vi "Initialize Variables.vi"(5 "subkey":string="Software\\DuPont\\BIMS", 6 "errorIN":errorcluster, 9 "InitCluster":cluster{"deployment":refnum<vi>}) -> (0 "errorOUT":errorcluster)   [LabVIEW 2010]
uses:
  <vilib>/registry/registry.llb/Registry SAM.ctl
  <vilib>/registry/registry.llb/Registry RtKey.ctl
panel:
  in  "DataFolder":refnum<vi>
  in  "Keys":enum16{"Root"}(ring)
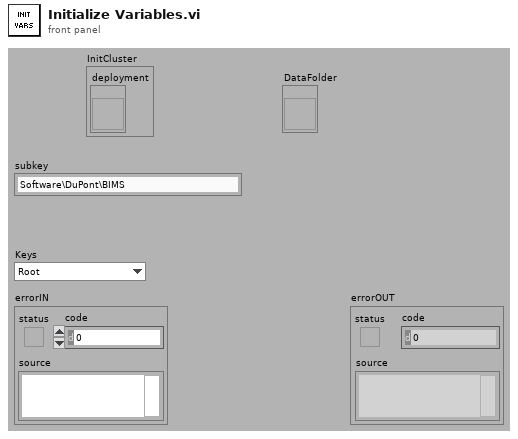
[diagram p1: front panel]
types:
  T1 = typedef "Registry SAM.ctl" = enum32{"KEY_QUERY_VALUE", "KEY_SET_VALUE", "KEY_CREATE_SUB_KEY", "KEY_ENUMERATE_SUB_KEYS", "KEY_NOTIFY", "KEY_CREATE_LINK", "KEY_READ", "KEY_WRITE", "KEY_ALL_ACCESS", "KEY_READ | KEY_WRITE"}
  T2 = typedef "Registry RtKey.ctl" = enum32{"HKEY_CLASSES_ROOT", "HKEY_CURRENT_USER", "HKEY_LOCAL_MACHINE", "HKEY_USERS", "HKEY_PERFORMANCE_DATA", "HKEY_CURRENT_CONFIG", "HKEY_DYN_DATA"}
  T3 = typedef "Registry refnum.ctl" = refnum<k1>
  T4 = cluster{"numValues":i32, "maxValueNameLen":i32, "maxValueDataLen":i32}
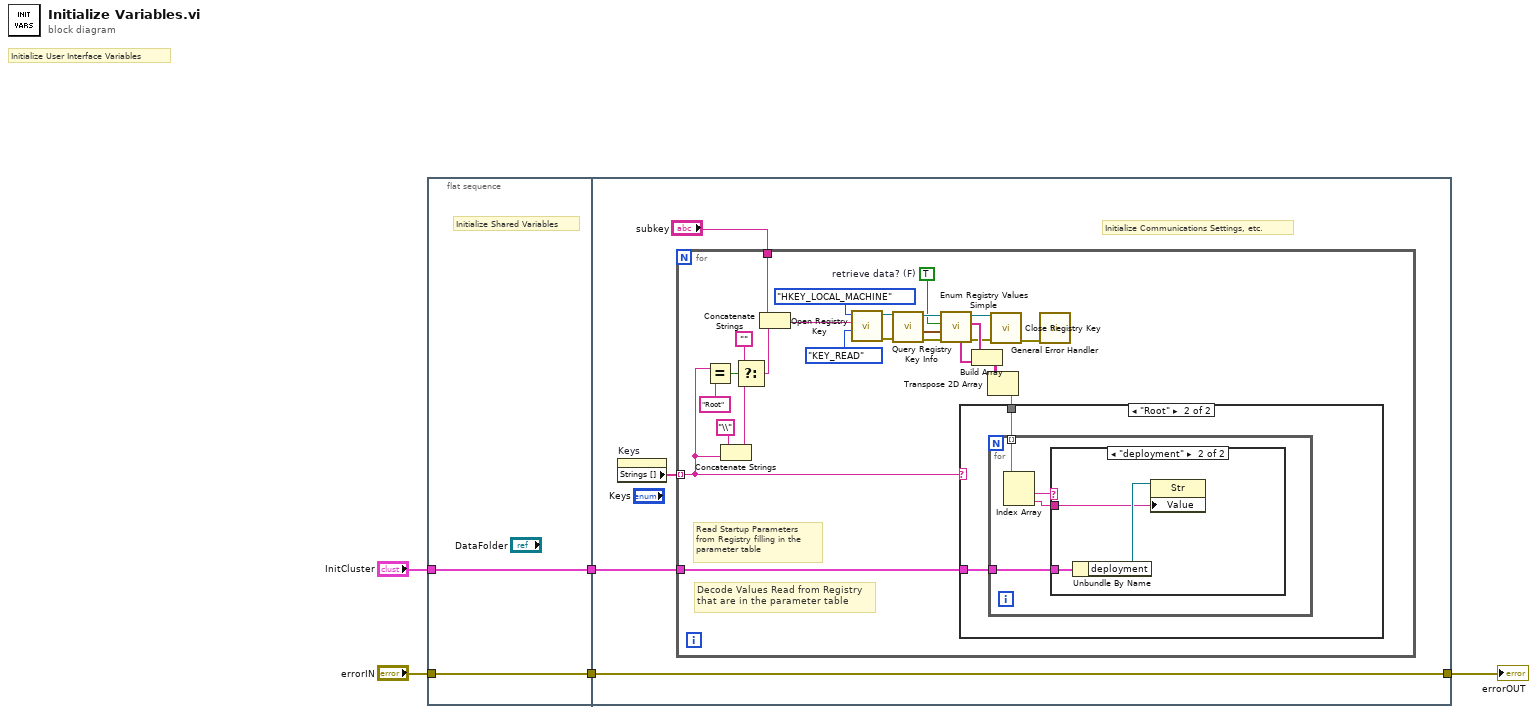
[diagram p0: block diagram]
diagram:
  # "Initialize User Interface Variables"
  n1 = flat-sequence {
    tunnel: [w7] -> w4
    tunnel: "errorIN" -> [w7]
    tunnel: "InitCluster" -> [w6]
    tunnel: [w6] -> w2
    tunnel: w4 -> [w10]
    tunnel: [w10] -> w3
    tunnel: w2 -> [w8]
    frame #0 {
      # "Initialize Shared Variables"
    }
    frame #1 {
      # "Initialize Communications Settings, etc."
      n2 = property on="Keys" class="Enum (strict)"() -> ("Strings []"=w9:string[])  [unwired: 2 in, 2 out]
      n3 = for {
        tunnel: "subkey" -> [w32]
        tunnel: w9 -> [w12] mode=indexing
        tunnel: w8 -> [w13]
        w24 = TRUE  # retrieve data? (F)
        # "Decode Values Read from Registry that are in the parameter table"
        # "Read Startup Parameters\nfrom Registry filling in the \nparameter table"
        n4 = Equal?(x=w12, y="Root" ("subkey")) -> (x = y?=w18:bool)
        n5 = Concatenate Strings("\\" ("subkey"), w12) -> (w15:string)
        n6 = Select(t="", s=w18, f=w15) -> (s? t:f=w17:string)
        n7 = Concatenate Strings(w32, w17) -> (w33:string)
        n8 = call <vilib>:"Open Registry Key.vi"("security access mask (KEY_READ | KEY_WRITE)"=Registry_SAM."KEY_READ", "subkey"=w33, "root key (HKEY_LOCAL_MACHINE)"=Registry_RtKey."HKEY_LOCAL_MACHINE") -> ("error out"=w29:errorcluster, "refnum out"=w28:T3)  [unwired: 1 in, 6 out]
        n9 = call <vilib>:"Query Registry Key Info.vi"("error in (no error)"=w29, "refnum"=w28) -> ("error out"=w27:errorcluster, "value info"=w26:T4, "refnum out"=w25:T3)  [unwired: 7 out]
        n10 = call <vilib>:"Enum Registry Values Simple.vi"("error in (no error)"=w27, "value info"=w26, "retrieve data? (F)"=w24, "refnum"=w25) -> ("error out"=w23:errorcluster, "values"=w35:string[], "refnum out"=w22:T3, "String/Binary data"=w21:string[])  [unwired: 4 out]
        n11 = Build Array(w35, w21) -> (w20:string[][])
        n12 = Transpose 2D Array(2D array=w20) -> (transposed array=w34:string[][])
        n13 = case shown="\"Root\"" w12 {
          tunnel: w34 -> [_ w38]
          tunnel: w13 -> [_ w37]
          frame Default {
          }
          frame "Root" {
            n14 = for {
              tunnel: w38 -> [w41] mode=indexing
              tunnel: w37 -> [w39]
              n15 = Index Array(array=w41) -> (element #1=w40:string, element #2=w42:string)  [unwired: 2 in]
              n16 = case shown="\"deployment\"" w40 {
                tunnel: w42 -> [_ w43]
                tunnel: w39 -> [_ w45]
                frame Default {
                }
                frame "deployment" {
                  n17 = Unbundle By Name(w45) -> ("deployment"=w44:refnum<vi>)
                  n18 = property class="Str"(reference=w44, "Value"=w43) -> ()  [unwired: 1 in, 2 out]
                }
              }
            }
          }
        }
        n19 = call <vilib>:"Close Registry Key.vi"("error in (no error)"=w23, "refnum"=w22) -> ("error out"=w36:errorcluster)  [unwired: 5 out]
        n20 = call <vilib>:"General Error Handler.vi"("error in (no error)"=w36) -> ()  [unwired: 10 in, 5 out]
      }
    }
  }
  "errorOUT" <- w3
